vi "Get Event Data In.vi"(8 "error in (no error)":errorcluster, 10 "Event Data Names":string[](array[string]), 11 "Diagram in":refnum<vi>) -> (0 "error out":errorcluster, 2 "OutputTerms[]":refnum<vi>[](array[refnum]), 3 "Diagram out":refnum<vi>)   [LabVIEW 2015, in "Scripting.lvlib"]
uses:
  Scripting.lvlib
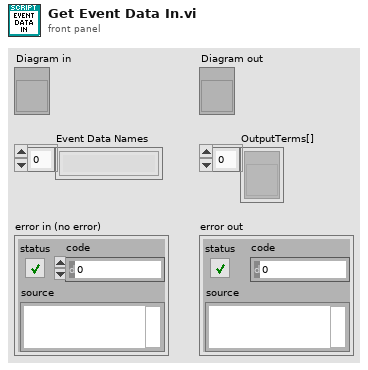
[diagram p1: front panel]
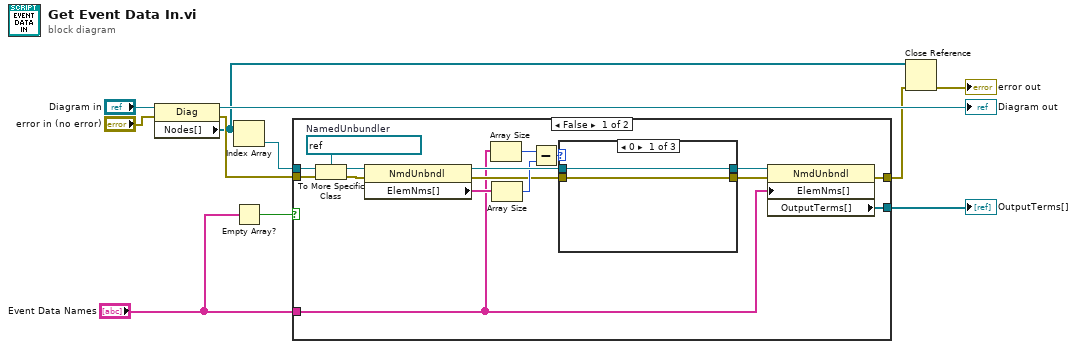
[diagram p0: block diagram]
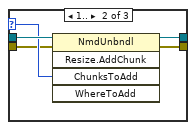
[diagram p2: hidden frame]
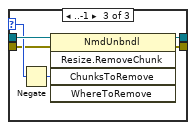
[diagram p3: hidden frame]
diagram:
  n1 = property class="Diag"(reference="Diagram in", error in="error in (no error)") -> (reference out=→"Diagram out":refnum<vi>, error out=w8:errorcluster, "Nodes[]"=w3:refnum<vi>[])
  n2 = Index Array(array=w3) -> (element=w7:refnum<vi>)  [unwired: 1 in]
  n3 = Empty Array?(array="Event Data Names") -> (empty?=w10:bool)
  n4 = case shown="False" w10 {
    tunnel: w7 -> [w27 _]
    tunnel: w8 -> [w26 w41]
    tunnel: "Event Data Names" -> [w12 _]
    tunnel: [w19 w41] -> w1
    tunnel: [w20 _] -> w11
    frame False {
      w25 = refnum<vi> refnum  # NamedUnbundler
      n5 = To More Specific Class(target class=w25, reference=w27, error in=w26) -> (specific class reference=w17:refnum<vi>, error out=w14:errorcluster)
      n6 = property class="NmdUnbndl"(reference=w17, error in=w14) -> (reference out=w24:refnum<vi>, error out=w13:errorcluster, "ElemNms[]"=w23:string[])
      n7 = Array Size(array=w12) -> (size(s)=w21:i32)
      n8 = Array Size(array=w23) -> (size(s)=w22:i32)
      n9 = Subtract(x=w21, y=w22) -> (x-y=w18:i32)
      n10 = case shown="0" w18 {
        selector: w18 -> [_ w33 w39]
        tunnel: w24 -> [w29 w34 w40]
        tunnel: [w29 w32 w38] -> w16
        tunnel: w13 -> [w28 w31 w36]
        tunnel: [w28 w30 w37] -> w15
        frame 0 {
        }
        frame 1.. {
          n11 = invoke class="NmdUnbndl" method="Resize.AddChunk"(reference=w34, error in=w31, "ChunksToAdd"=w33) -> (reference out=w32:refnum<vi>, error out=w30:errorcluster)  [unwired: 2 in, 3 out]
        }
        frame ..-1 {
          n12 = Negate(x=w39) -> (-x=w35:i32)
          n13 = invoke class="NmdUnbndl" method="Resize.RemoveChunk"(reference=w40, error in=w36, "ChunksToRemove"=w35) -> (reference out=w38:refnum<vi>, error out=w37:errorcluster)  [unwired: 2 in, 3 out]
        }
      }
      n14 = property class="NmdUnbndl"(reference=w16, error in=w15, "ElemNms[]"=w12) -> (error out=w19:errorcluster, "OutputTerms[]"=w20:refnum<vi>[])  [unwired: 1 out]
    }
    frame True {
    }
  }
  "OutputTerms[]" <- w11
  n15 = Close Reference(reference=w3, error in (no error)=w1) -> (error out=→"error out":errorcluster)
